vi "ArrayOfPathComponentStrings.vi"(1 "PathStringIn":string) -> (0 "ArrayOfPathComponentStringsOut":string[](array[string]))   [LabVIEW 2015]
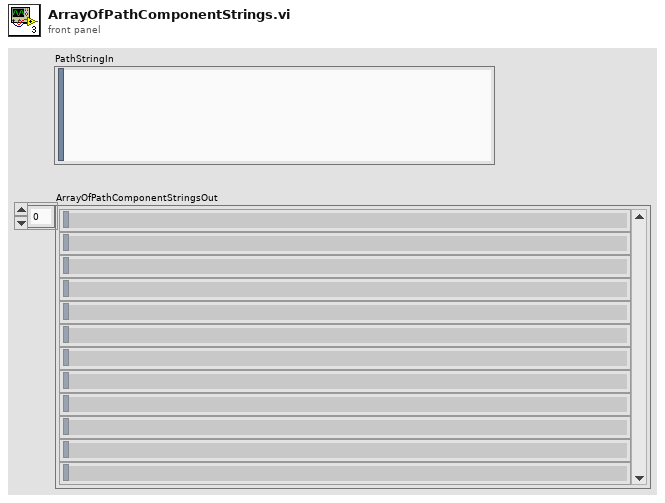
[diagram p1: front panel]
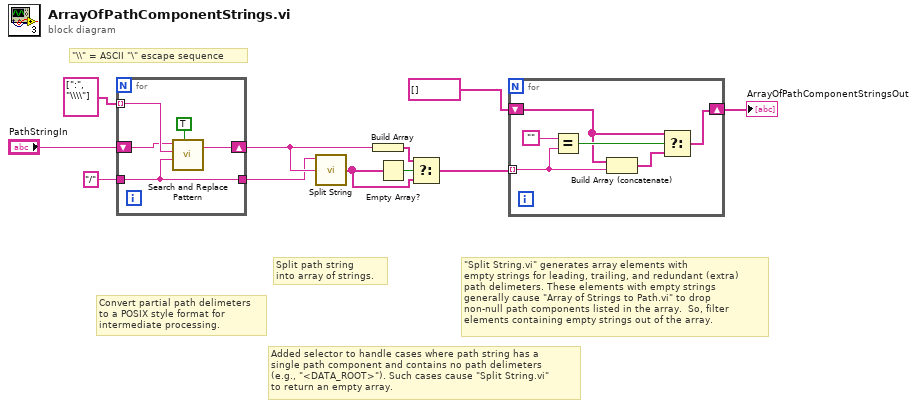
[diagram p0: block diagram]
diagram:
  # "Added selector to handle cases where path string has a \nsingle path component and contains no path delimeters\n(e.g., \"<DATA_ROOT>\"). Such cases cause \"Split String.vi\"\nto return an empty array."
  # "\"Split String.vi\" generates array elements with\nempty strings for leading, trailing, and redundant (extra)\npath delimeters. These elements with empty strings \ngenerally cause \"Array of Strings to Path.vi\" to drop \nnon-null path components listed in the array.  So, filter\nelements containing empty strings out of the array."
  # "Split path string\ninto array of strings."
  # "Convert partial path delimeters\nto a POSIX style format for\nintermediate processing."
  # "\"\\\\\" = ASCII \"\\\" escape sequence"
  n1 = for {
    tunnel: string[] [":", "\\\\"] -> [w16] mode=indexing
    shift-right: [w14] -> w9
    shift-left: "PathStringIn" -> [w13]
    tunnel: "/" ("replace string (\"\")") -> [w12]
    tunnel: [w12] -> w1
    n2 = call <vilib>:"Search and Replace Pattern.vi"("string"=w13, "regular expression (\"\")"=w16, "replace string (\"\")"=w12, "replace all? (F)"=TRUE) -> ("result string"=w14:string)  [unwired: 1 in, 1 out]
  }
  n3 = call <vilib>:"Split String.vi"("Split Pattern"=w1, "Input String"=w9) -> ("Split String"=w7:string[])  [unwired: 5 in]
  n4 = Build Array(w9) -> (w8:string[])
  n5 = Empty Array?(array=w7) -> (empty?=w6:bool)
  n6 = Select(t=w8, s=w6, f=w7) -> (s? t:f=w11:string[])
  n7 = for {
    shift-right: [w20] -> w2
    shift-left: string[] [] -> [w19]
    tunnel: w11 -> [w18] mode=indexing
    n8 = Equal?(x="", y=w18) -> (x = y?=w21:bool)
    n9 = Build Array (concatenate)(w19, w18) -> (w17:string[])
    n10 = Select(t=w19, s=w21, f=w17) -> (s? t:f=w20:string[])
  }
  "ArrayOfPathComponentStringsOut" <- w2
